vi "Circle Test.vi"() -> ()   [LabVIEW 2019]
uses:
  Classes/Controller/Controller.lvclass
  Drivers/Aerotech A3200/Aerotech VIs.lvlib
panel:
  in  "stop":bool
  in  "Go":bool
  in  "Direction":u16(ring) items=["Clockwise", "Counter-clockwise"]
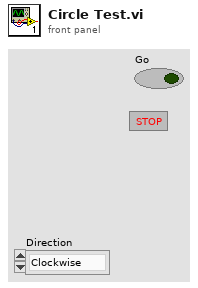
[diagram p1: front panel]
types:
  T1 = typedef "Controller.lvclass/Controllers.ctl" = cluster{"I-O.lvclass":refnum<class "I-O.lvclass">, "Dispenser.lvclass":refnum<class "Dispenser.lvclass">, "Gantry":refnum<k24>}
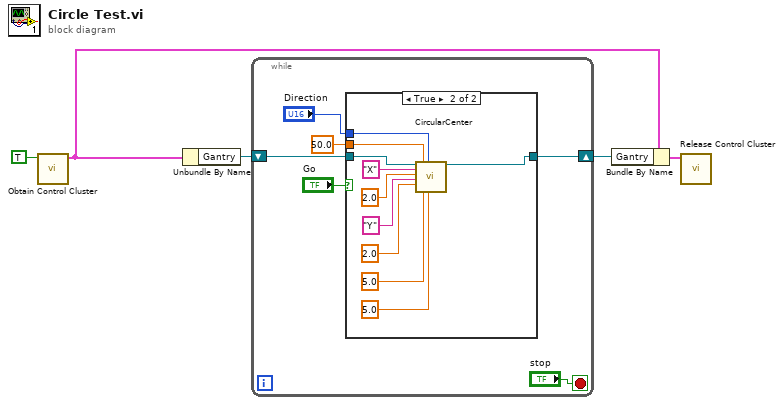
[diagram p0: block diagram]
diagram:
  n1 = call "Obtain Control Cluster.vi"("Motion"=TRUE) -> ("Control Out"=w3:T1)  [unwired: 10 in]
  n2 = Unbundle By Name(w3) -> ("Gantry"=w2:refnum<k24>)
  n3 = while {
    shift-right: [w9] -> w5
    shift-left: w2 -> [w6]
    stop <- "stop" stop-if-true
    n4 = case shown="True" "Go" {
      tunnel: w6 -> [w12 w22]
      tunnel: 50.0 ("Speed") -> [_ w19]
      tunnel: "Direction" -> [_ w20]
      tunnel: [w12 w21] -> w9
      frame False {
      }
      frame True {
        n5 = call "CircularCenter.vi"("controller in"=w22, "axis 1 name"="X", "axis 1 endpoint"=2.0, "axis 2 name"="Y", "axis 2 endpoint"=2.0, "speed"=w19, "axis 1 center point"=5.0, "direction"=w20, "axis 2 center point"=5.0) -> ("controller out"=w21:refnum<k24>)  [unwired: 9 in, 1 out]
      }
    }
  }
  n6 = Bundle By Name(cluster=w3, "Gantry"=w5) -> (w4:T1)
  n7 = call "Release Control Cluster.vi"("output cluster"=w4) -> ()  [unwired: 11 in]
